vi "Func-엑셀 데이터를 그래프로 출력.vi"() -> ()   [LabVIEW 2015] (continued)
\t65\t69.654\n65\t65\t69.656\n65\t65\t69.657\n65\t65\t69.656\n65\t65\t69.656\n65\t65\t69.657\n65\t65\t69.658\n65\t65\t69.662\n65\t65\t69.662\n65\t65\t69.666\n65\t65\t69.667\n65\t65\t69.667\n65\t65\t69.668\n65\t65\t69.664\n65\t65\t69.666\n65\t65\t69.667\n65\t65\t69.671\n65\t65\t69.671\n65\t65\t69.671\n65\t65\t69.672\n65\t65\t69.675\n65\t65\t69.676\n65\t65\t69.675\n65\t65\t69.681\n65\t65\t69.685\n65\t65\t69.686\n65\t65\t69.688\n65\t65\t69.689\n65\t65\t69.69\n65\t65\t69.687\n65\t65\t69.687\n65\t65\t69.693\n65\t65\t69.694\n65\t65\t69.694\n65\t65\t69.696\n65\t65\t69.696\n65\t65\t69.699\n65\t65\t69.697\n65\t65\t69.696\n65\t65\t69.699\n65\t65\t69.695\n65\t65\t69.694\n65\t65\t69.693\n65\t65\t69.696\n65\t65\t69.698\n65\t65\t69.7\n65\t65\t69.707\n65\t65\t69.712\n65\t65\t69.717\n65\t65\t69.718\n65\t65\t69.72\n65\t65\t69.72\n65\t65\t69.719\n65\t65\t69.72\n65\t65\t69.721\n65\t65\t69.721\n65\t65\t69.722\n65\t65\t69.718\n65\t65\t69.721\n65\t65\t69.721\n65\t65\t69.719\n65\t65\t69.719\n65\t65\t69.718\n65\t65\t69.721\n65\t65\t69.725\n65\t65\t69.727\n65\t65\t69.73\n65\t65\t69.73\n65\t65\t69.73\n65\t65\t69.736\n65\t65\t69.736\n65\t65\t69.737\n65\t65\t69.739\n65\t65\t69.744\n65\t65\t69.746\n65\t65\t69.742\n65\t65\t69.743\n65\t65\t69.742\n65\t65\t69.746\n65\t65\t69.742\n65\t65\t69.746\n65\t65\t69.747\n65\t65\t69.751\n65\t65\t69.755\n65\t65\t69.755\n65\t65\t69.757\n65\t65\t69.761\n65\t65\t69.766\n65\t65\t69.764\n65\t65\t69.765\n65\t65\t69.763\n65\t65\t69.77\n65\t65\t69.771\n65\t65\t69.769\n65\t65\t69.773\n65\t65\t69.769\n65\t65\t69.771\n65\t65\t69.769\n65\t65\t69.766\n65\t65\t69.768\n65\t65\t69.768\n65\t65\t69.77\n65\t65\t69.772\n65\t65\t69.773\n65\t65\t69.773\n65\t65\t69.772\n65\t65\t69.773\n65\t65\t69.779\n65\t65\t69.78\n65\t65\t69.781\n65\t65\t69.786\n65\t65\t69.79\n65\t65\t69.793\n65\t65\t69.791\n65\t65\t69.789\n65\t65\t69.787\n65\t65\t69.788\n65\t65\t69.786\n65\t65\t69.784\n65\t65\t69.788\n65\t65\t69.79\n65\t65\t69.791\n65\t65\t69.79\n65\t65\t69.79\n65\t65\t69.792\n65\t65\t69.791\n65\t65\t69.789\n65\t65\t69.79\n65\t65\t69.795\n65\t65\t69.798\n65\t65\t69.8\n65\t65\t69.804\n65\t65\t69.806\n65\t65\t69.805\n65\t65\t69.803\n65\t65\t69.806\n65\t65\t69.806\n65\t65\t69.804\n65\t65\t69.808\n65\t65\t69.809\n65\t65\t69.81\n65\t65\t69.807\n65\t65\t69.809\n65\t65\t69.812\n65\t65\t69.811\n65\t65\t69.813\n65\t65\t69.816\n65\t65\t69.82\n65\t65\t69.821\n65\t65\t69.82\n65\t65\t69.823\n65\t65\t69.823\n65\t65\t69.826\n65\t65\t69.823\n65\t65\t69.824\n65\t65\t69.828\n65\t65\t69.832\n65\t65\t69.835\n65\t65\t69.833\n65\t65\t69.838\n65\t65\t69.838\n65\t65\t69.836\n65\t65\t69.833\n65\t65\t69.836\n65\t65\t69.836\n65\t65\t69.839\n65\t65\t69.843\n65\t65\t69.844\n65\t65\t69.85\n65\t65\t69.846\n65\t65\t69.847\n65\t65\t69.844\n65\t65\t69.845\n65\t65\t69.848\n65\t65\t69.844\n65\t65\t69.848\n65\t65\t69.852\n65\t65\t69.857\n65\t65\t69.855\n65\t65\t69.855\n65\t65\t69.86\n65\t65\t69.861\n65\t65\t69.857\n65\t65\t69.857\n65\t65\t69.859\n65\t65\t69.858\n65\t65\t69.856\n65\t65\t69.855\n65\t65\t69.856\n65\t65\t69.854\n65\t65\t69.854\n65\t65\t69.855\n65\t65\t69.858\n65\t65\t69.863\n65\t65\t69.868\n65\t65\t69.87\n65\t65\t69.873\n65\t65\t69.877\n65\t65\t69.875\n65\t65\t69.878\n65\t65\t69.879\n65\t65\t69.879\n65\t65\t69.877\n65\t65\t69.877\n65\t65\t69.877\n65\t65\t69.875\n65\t65\t69.874\n65\t65\t69.876\n65\t65\t69.877\n65\t65\t69.879\n65.083\t65.06\t70.457\n65.167\t65.12\t70.467\n65.25\t65.04\t70.467\n65.333\t64.94\t70.484\n65.417\t64.87\t70.475\n65.5\t64.77\t70.48\n65.583\t64.66\t70.477\n65.667\t64.54\t70.491\n65.75\t64.44\t70.489\n65.833\t64.34\t70.495\n65.917\t64.26\t70.497\n66\t64.18\t70.494\n66.083\t64.15\t70.494\n66.167\t64.12\t70.506\n66.25\t64.13\t70.493\n66.333\t64.15\t70.499\n66.417\t64.19\t70.495\n66.5\t64.25\t70.502\n66.583\t64.33\t70.495\n66.667\t64.42\t70.505\n66.75\t64.52\t70.501\n66.833\t64.63\t70.495\n66.917\t64.76\t70.491\n67\t64.89\t70.501\n67.083\t65.01\t70.506\n67.167\t65.14\t70.499\n67.25\t65.27\t70.494\n67.333\t65.4\t70.482\n67.417\t65.52\t70.498\n67.5\t65.64\t70.502\n67.583\t65.75\t70.504\n67.667\t65.85\t70.494\n67.75\t65.94\t70.503\n67.833\t66.03\t70.493\n67.917\t66.12\t70.498\n68\t66.21\t70.496\n68.083\t66.3\t70.507\n68.167\t66.38\t70.51\n68.25\t66.44\t70.51\n68.333\t66.52\t70.518\n68.417\t66.6\t70.514\n68.5\t66.67\t70.516\n68.583\t66.74\t70.525\n68.667\t66.81\t70.535\n68.75\t66.88\t70.533\n68.833\t66.95\t70.542\n68.917\t67.02\t70.544\n69\t67.1\t70.551\n69.083\t67.17\t70.559\n69.167\t67.24\t70.577\n69.25\t67.32\t70.583\n69.333\t67.4\t70.588\n69.417\t67.48\t70.612\n69.5\t67.56\t70.616\n69.583\t67.65\t70.624\n69.667\t67.73\t70.634\n69.75\t67.82\t70.644\n69.833\t67.9\t70.655\n69.917\t67.99\t70.665\n70\t68.07\t70.691\n70.083\t68.16\t70.706\n70.167\t68.25\t70.709\n70.25\t68.33\t70.732\n70.333\t68.41\t70.75\n70.417\t68.49\t70.766\n70.5\t68.57\t70.788\n70.583\t68.65\t70.798\n70.667\t68.72\t70.818\n70.75\t68.79\t70.832\n70.833\t68.87\t70.861\n70.917\t68.94\t70.886\n71\t69.01\t70.899\n71.083\t69.08\t70.924\n71.167\t69.15\t70.942\n71.25\t69.23\t70.965\n71.333\t69.31\t70.995\n71.417\t69.4\t71.013\n71.5\t69.47\t71.041\n71.583\t69.55\t71.06\n71.667\t69.63\t71.091\n71.75\t69.72\t71.109\n71.833\t69.79\t71.137\n71.917\t69.87\t71.155\n72\t69.96\t71.191\n72.083\t70.04\t71.219\n72.167\t70.12\t71.246\n72.25\t70.21\t71.273\n72.333\t70.28\t71.305\n72.417\t70.35\t71.341\n72.5\t70.43\t71.368\n72.583\t70.52\t71.398\n72.667\t70.6\t71.431\n72.75\t70.68\t71.465\n72.833\t70.75\t71.491\n72.917\t70.85\t71.529\n73\t70.95\t71.562\n73.083\t71.03\t71.589\n73.167\t71.1\t71.629\n73.25\t71.18\t71.661\n73.333\t71.26\t71.695\n73.417\t71.35\t71.732\n73.5\t71.44\t71.762\n73.583\t71.51\t71.796\n73.667\t71.6\t71.842\n73.75\t71.68\t71.891\n73.833\t71.77\t71.914\n73.917\t71.85\t71.955\n74\t71.95\t71.99\n74.083\t72.03\t72.033\n74.167\t72.12\t72.076\n74.25\t72.2\t72.118\n74.333\t72.28\t72.155\n74.417\t72.36\t72.19\n74.5\t72.45\t72.229\n74.583\t72.54\t72.275\n74.667\t72.62\t72.317\n74.75\t72.71\t72.354\n74.833\t72.79\t72.4\n74.917\t72.88\t72.451\n75\t72.97\t72.485\n75.083\t73.05\t72.525\n75.167\t73.14\t72.57\n75.25\t73.23\t72.625\n75.333\t73.32\t72.676\n75.417\t73.39\t72.714\n75.5\t73.48\t72.757\n75.583\t73.56\t72.803\n75.667\t73.64\t72.859\n75.75\t73.71\t72.902\n75.833\t73.8\t72.946\n75.917\t73.87\t72.994\n76\t73.95\t73.047\n76.083\t74.04\t73.093\n76.167\t74.12\t73.138\n76.25\t74.19\t73.19\n76.333\t74.29\t73.231\n76.417\t74.36\t73.286\n76.5\t74.43\t73.338\n76.583\t74.5\t73.391\n76.667\t74.58\t73.448\n76.75\t74.67\t73.487\n76.833\t74.73\t73.552\n76.917\t74.81\t73.599\n77\t74.89\t73.645\n77.083\t74.96\t73.697\n77.167\t75.03\t73.747\n77.25\t75.13\t73.803\n77.333\t75.22\t73.861\n77.417\t75.31\t73.913\n77.5\t75.39\t73.964\n77.583\t75.47\t74.02\n77.667\t75.56\t74.083\n77.75\t75.64\t74.129\n77.833\t75.75\t74.178\n77.917\t75.83\t74.235\n78\t75.92\t74.289\n78.083\t76.01\t74.354\n78.167\t76.09\t74.406\n78.25\t76.19\t74.462\n78.333\t76.27\t74.521\n78.417\t76.36\t74.575\n78.5\t76.44\t74.633\n78.583\t76.53\t74.685\n78.667\t76.61\t74.745\n78.75\t76.7\t74.807\n78.833\t76.78\t74.876\n78.917\t76.86\t74.925\n79\t76.93\t74.988\n79.083\t77.01\t75.031\n79.167\t77.1\t75.092\n79.25\t77.17\t75.159\n79.333\t77.25\t75.212\n79.417\t77.32\t75.278\n79.5\t77.38\t75.335\n79.583\t77.46\t75.405\n79.667\t77.55\t75.454\n79.75\t77.63\t75.521\n79.833\t77.7\t75.579\n79.917\t77.78\t75.64\n80\t77.87\t75.699\n80.083\t77.95\t75.763\n80.167\t78.04\t75.835\n80.25\t78.13\t75.897\n80.333\t78.21\t75.958\n80.417\t78.28\t76.013\n80.5\t78.35\t76.079\n80.583\t78.42\t76.156\n80.667\t78.51\t76.198\n80.75\t78.59\t76.271\n80.833\t78.66\t76.334\n80.917\t78.74\t76.404\n81\t78.82\t76.461\n81.083\t78.9\t76.53\n81.167\t78.99\t76.588\n81.25\t79.08\t76.653\n81.333\t79.16\t76.718\n81.417\t79.23\t76.778\n81.5\t79.32\t76.851\n81.583\t79.4\t76.918\n81.667\t79.49\t76.985\n81.75\t79.57\t77.039\n81.833\t79.65\t77.109\n81.917\t79.74\t77.178\n82\t79.81\t77.242\n82.083\t79.91\t77.295\n82.167\t79.99\t77.368\n82.25\t80.08\t77.443\n82.333\t80.15\t77.496\n82.417\t80.24\t77.565\n82.5\t80.33\t77.635\n82.583\t80.41\t77.704\n82.667\t80.48\t77.763\n82.75\t80.56\t77.827\n82.833\t80.66\t77.901\n82.917\t80.74\t77.966\n83\t80.81\t78.036\n83.083\t80.9\t78.098\n83.167\t80.99\t78.164\n83.25\t81.06\t78.234\n83.333\t81.14\t78.297\n83.417\t81.22\t78.361\n83.5\t81.31\t78.441\n83.583\t81.4\t78.506\n83.667\t81.49\t78.576\n83.75\t81.57\t78.64\n83.833\t81.66\t78.698\n83.917\t81.73\t78.78\n84\t81.81\t78.841\n84.083\t81.89\t78.913\n84.167\t81.96\t78.985\n84.25\t82.04\t79.053\n84.333\t82.11\t79.114\n84.417\t82.17\t79.187\n84.5\t82.26\t79.259\n84.583\t82.35\t79.32\n84.667\t82.43\t79.391\n84.75\t82.51\t79.466\n84.833\t82.6\t79.528\n84.917\t82.69\t79.601\n85\t82.76\t79.662\n85\t82.77\t79.665\n85\t82.78\t79.667\n85\t82.79\t79.671\n85\t82.8\t79.673\n85\t82.81\t79.68\n85\t82.82\t79.688\n85\t82.82\t79.696\n85\t82.82\t79.709\n85\t82.83\t79.716\n85\t82.84\t79.724\n85\t82.85\t79.737\n85\t82.86\t79.741\n85\t82.86\t79.747\n85\t82.87\t79.755\n85\t82.88\t79.764\n85\t82.89\t79.775\n85\t82.9\t79.783\n85\t82.91\t79.791\n85\t82.91\t79.801\n85\t82.92\t79.808\n85\t82.93\t79.813\n85\t82.93\t79.818\n85\t82.94\t79.826\n85\t82.95\t79.831\n85\t82.96\t79.835\n85\t82.97\t79.84\n85\t82.97\t79.845\n85\t82.98\t79.854\n85\t82.99\t79.855\n85\t83\t79.863\n85\t83.01\t79.874\n85\t83.02\t79.879\n85\t83.03\t79.883\n85\t83.03\t79.896\n85\t83.04\t79.91\n85\t83.04\t79.913\n85\t83.05\t79.921\n85\t83.06\t79.928\n85\t83.07\t79.933\n85\t83.07\t79.941\n85\t83.08\t79.945\n85\t83.09\t79.954\n85\t83.1\t79.961\n85\t83.11\t79.967\n85\t83.12\t79.974\n85\t83.13\t79.975\n85\t83.14\t79.981\n85\t83.14\t79.99\n85\t83.15\t79.994\n85\t83.15\t80.003\n85\t83.15\t80.014\n85\t83.15\t80.022\n85\t83.16\t80.028\n85\t83.17\t80.038\n85\t83.18\t80.048\n85\t83.19\t80.052\n85\t83.2\t80.064\n85\t83.2\t80.071\n85\t83.21\t80.078\n85\t83.21\t80.082\n85\t83.22\t80.085\n85\t83.22\t80.096\n85\t83.23\t80.098\n85\t83.23\t80.104\n85\t83.24\t80.113\n85\t83.24\t80.118\n85\t83.25\t80.125\n85\t83.25\t80.132\n85\t83.25\t80.139\n85\t83.25\t80.146\n85\t83.26\t80.159\n85\t83.27\t80.165\n85\t83.27\t80.17\n85\t83.28\t80.183\n85\t83.29\t80.189\n85\t83.29\t80.196\n85\t83.3\t80.199\n85\t83.3\t80.208\n85\t83.31\t80.214\n85\t83.31\t80.217\n85\t83.32\t80.221\n85\t83.33\t80.229\n85\t83.33\t80.234\n85\t83.34\t80.242\n85\t83.35\t80.252\n85\t83.36\t80.259\n85\t83.36\t80.268\n85\t83.36\t80.274\n85\t83.36\t80.281\n85\t83.36\t80.286\n85\t83.37\t80.291\n85\t83.38\t80.298\n85\t83.39\t80.304\n85\t83.39\t80.315\n85\t83.4\t80.319\n85\t83.41\t80.331\n85\t83.41\t80.337\n85\t83.41\t80.343\n85\t83.42\t80.35\n85\t83.42\t80.355\n85\t83.43\t80.365\n85\t83.44\t80.371\n85\t83.45\t80.377\n85\t83.45\t80.386\n85\t83.46\t80.395\n85\t83.46\t80.401\n85\t83.47\t80.405\n85\t83.47\t80.416\n85\t83.47\t80.427\n85\t83.47\t80.429\n85\t83.47\t80.434\n85\t83.47\t80.442\n85\t83.48\t80.455\n85\t83.48\t80.456\n85\t83.49\t80.459\n85\t83.5\t80.473\n85\t83.5\t80.481\n85\t83.5\t80.488\n85\t83.51\t80.494\n85\t83.52\t80.502\n85\t83.52\t80.509\n85\t83.53\t80.516\n85\t83.54\t80.518\n85\t83.54\t80.522\n85\t83.55\t80.527\n85\t83.55\t80.536\n85\t83.56\t80.54\n85\t83.57\t80.548\n85\t83.58\t80.56\n85\t83.58\t80.568\n85\t83.58\t80.575\n85\t83.58\t80.58\n85\t83.59\t80.591\n85\t83.59\t80.594\n85\t83.6\t80.599\n85\t83.61\t80.607\n85\t83.61\t80.619\n85\t83.62\t80.624\n85\t83.63\t80.63\n85\t83.64\t80.636\n85\t83.65\t80.639\n85\t83.65\t80.646\n85\t83.66\t80.649\n85\t83.67\t80.655\n85\t83.68\t80.667\n85\t83.68\t80.676\n85\t83.69\t80.684\n85\t83.69\t80.694\n85\t83.69\t80.702\n85\t83.69\t80.712\n85\t83.69\t80.716\n85\t83.7\t80.72\n85\t83.71\t80.729\n85\t83.71\t80.735\n85\t83.72\t80.736\n85\t83.73\t80.741\n85\t83.73\t80.748\n85\t83.74\t80.754\n85\t83.75\t80.764\n85\t83.75\t80.771\n85\t83.76\t80.782\n85\t83.77\t80.793\n85\t83.77\t80.801\n85\t83.78\t80.811\n85\t83.79\t80.815\n85\t83.8\t80.82\n85\t83.8\t80.826\n85\t83.8\t80.834\n85\t83.81\t80.84\n85\t83.82\t80.845\n85\t83.82\t80.852\n85\t83.83\t80.859\n85\t83.84\t80.864\n85\t83.84\t80.871\n85\t83.85\t80.879\n85\t83.86\t80.888\n85\t83.87\t80.895\n85\t83.88\t80.9\n85\t83.89\t80.91\n85\t83.89\t80.919\n85\t83.9\t80.921\n85\t83.91\t80.93\n85\t83.91\t80.936\n85\t83.91\t80.944\n85\t83.92\t80.953\n85\t83.93\t80.958\n85\t83.94\t80.967\n85\t83.95\t80.974\n85\t83.95\t80.982\n85\t83.96\t80.987\n85\t83.97\t80.993\n85\t83.98\t80.996\n85\t83.99\t81.004\n85\t84\t81.007\n85\t84\t81.013\n85\t84.01\t81.023\n85\t84.01\t81.032\n85\t84.02\t81.038\n85\t84.02\t81.054\n85\t84.03\t81.064\n85\t84.03\t81.071\n85\t84.04\t81.076\n85\t84.04\t81.083\n85\t84.05\t81.095\n85\t84.06\t81.097\n85\t84.06\t81.105\n85\t84.07\t81.111\n85\t84.08\t81.121\n85\t84.09\t81.126\n85\t84.09\t81.129\n85\t84.1\t81.133\n85\t84.11\t81.136\n85\t84.11\t81.146\n85\t84.12\t81.154\n85\t84.12\t81.157\n85\t84.12\t81.168\n85\t84.13\t81.177\n85\t84.14\t81.186\n85\t84.14\t81.193\n85\t84.15\t81.201\n85\t84.15\t81.213\n85\t84.16\t81.218\n85\t84.16\t81.226\n85\t84.17\t81.227\n85\t84.17\t81.232\n85\t84.18\t81.238\n85\t84.18\t81.246\n85\t84.19\t81.254\n85\t84.2\t81.261\n85\t84.2\t81.273\n85\t84.21\t81.282\n85\t84.22\t81.286\n85\t84.22\t81.292\n85\t84.23\t81.3\n85\t84.23\t81.303\n85\t84.23\t81.314\n85\t84.24\t81.319\n85\t84.24\t81.325\n85\t84.25\t81.336\n85\t84.25\t81.345\n85\t84.26\t81.35\n85\t84.26\t81.358\n85\t84.27\t81.364\n85\t84.28\t81.37\n85\t84.28\t81.378\n85\t84.29\t81.384\n85\t84.3\t81.398\n85\t84.3\t81.405\n85\t84.3\t81.416\n85\t84.31\t81.422\n85\t84.32\t81.427\n85\t84.32\t81.431\n85\t84.33\t81.436\n85\t84.34\t81.443\n85\t84.34\t81.442\n85\t84.34\t81.453\n85\t84.35\t81.457\n85\t84.36\t81.461\n85\t84.36\t81.466\n85\t84.37\t81.47\n85\t84.38\t81.479\n85\t84.38\t81.486\n85\t84.39\t81.491\n85\t84.39\t81.502\n85\t84.4\t81.509\n85\t84.41\t81.516\n85\t84.42\t81.523\n85\t84.43\t81.53\n85\t84.43\t81.539\n85\t84.44\t81.549\n85\t84.44\t81.555\n85\t84.45\t81.56\n85\t84.45\t81.566\n85\t84.45\t81.572\n85\t84.46\t81.579\n85\t84.46\t81.589\n85\t84.47\t81.6\n85\t84.47\t81.61\n85\t84.47\t81.617\n85\t84.48\t81.628\n85\t84.48\t81.629\n85\t84.49\t81.635\n85\t84.49\t81.638\n85\t84.5\t81.648\n85\t84.5\t81.657\n85\t84.51\t81.662\n85\t84.51\t81.676\n85\t84.51\t81.68\n85\t84.52\t81.687\n85\t84.52\t81.695\n85\t84.53\t81.7\n85\t84.53\t81.7\n85\t84.54\t81.705\n85\t84.55\t81.714\n85\t84.55\t81.722\n85\t84.55\t81.724\n85\t84.55\t81.729\n85\t84.56\t81.742\n85\t84.56\t81.748\n85\t84.56\t81.755\n85\t84.56\t81.764\n85\t84.57\t81.773\n85\t84.57\t81.776\n85\t84.57\t81.786\n85\t84.58\t81.789\n85\t84.58\t81.793\n85\t84.59\t81.8\n85\t84.59\t81.804\n85\t84.59\t81.81\n85\t84.59\t81.816\n85\t84.6\t81.829\n85\t84.6\t81.839\n85\t84.61\t81.849\n85\t84.61\t81.857\n85\t84.61\t81.871\n85\t84.61\t81.877\n85\t84.61\t81.881\n85\t84.61\t81.89\n85\t84.61\t81.893\n85\t84.62\t81.899\n85\t84.62\t81.909\n85\t84.62\t81.916\n85\t84.62\t81.92\n85\t84.63\t81.931\n85\t84.63\t81.934\n85\t84.63\t81.941\n85\t84.63\t81.948\n85\t84.64\t81.953\n85\t84.64\t81.962\n85\t84.64\t81.968\n85\t84.64\t81.978\n85\t84.64\t81.986\n85\t84.64\t81.993\n85\t84.65\t81.999\n85\t84.65\t82.005\n85\t84.65\t82.016\n85\t84.65\t82.018\n85\t84.65\t82.023\n85\t84.66\t82.03\n85\t84.66\t82.037\n85\t84.66\t82.043\n85\t84.66\t82.047\n85\t84.67\t82.058\n85\t84.67\t82.068\n85\t84.67\t82.075\n85\t84.67\t82.08\n85\t84.67\t82.089\n85\t84.67\t82.093\n85\t84.67\t82.098\n85\t84.67\t82.109\n85\t84.68\t82.114\n85\t84.68\t82.123\n85\t84.68\t82.13\n85\t84.69\t82.138\n85\t84.69\t82.144\n85\t84.69\t82.148\n85\t84.7\t82.153\n85\t84.7\t82.167\n85\t84.7\t82.173\n85\t84.7\t82.18\n85\t84.71\t82.191\n85\t84.71\t82.196\n85\t84.71\t82.203\n85\t84.71\t82.207\n85\t84.71\t82.213\n85\t84.72\t82.218\n85\t84.72\t82.226\n85\t84.72\t82.232\n85\t84.73\t82.238\n85\t84.73\t82.247\n85\t84.73\t82.253\n85\t84.74\t82.261\n85\t84.74\t82.266\n85\t84.74\t82.274\n85\t84.75\t82.285\n85\t84.75\t82.288\n85\t84.76\t82.291\n85\t84.76\t82.302\n85\t84.77\t82.307\n85\t84.77\t82.313\n85\t84.77\t82.314\n85\t84.77\t82.318\n85\t84.78\t82.326\n85\t84.78\t82.335\n85\t84.78\t82.343\n85\t84.78\t82.35\n85\t84.78\t82.363\n85\t84.78\t82.37\n85\t84.79\t82.379\n85\t84.8\t82.384\n85\t84.8\t82.39\n85\t84.8\t82.396\n85\t84.81\t82.405\n85\t84.81\t82.413\n85\t84.81\t82.422\n85\t84.81\t82.429\n85\t84.81\t82.435\n85\t84.82\t82.439\n85\t84.82\t82.449\n85\t84.82\t82.456\n85\t84.83\t82.458\n85\t84.83\t82.463\n85\t84.82\t82.467\n85\t84.83\t82.477\n85\t84.83\t82.484\n85\t84.83\t82.489\n85\t84.83\t82.501\n85\t84.84\t82.511\n85\t84.84\t82.519\n85\t84.84\t82.531\n85\t84.85\t82.533\n85\t84.85\t82.545\n85\t84.85\t82.552\n85\t84.85\t82.555\n85\t84.85\t82.567\n85\t84.86\t82.57\n85\t84.86\t82.577\n85\t84.86\t82.58\n85\t84.87\t82.581\n85\t84.87\t82.591\n85\t84.87\t82.594\n85\t84.88\t82.601\n85\t84.88\t82.604\n85\t84.88\t82.618\n85\t84.88\t82.628\n85\t84.88\t82.629\n85\t84.88\t82.638\n85\t84.88\t82.648\n85\t84.88\t82.658\n85\t84.88\t82.658\n85\t84.88\t82.666\n85\t84.88\t82.675\n85\t84.89\t82.682\n85\t84.9\t82.686\n85\t84.91\t82.688\n85\t84.92\t82.696\n85\t84.93\t82.701\n85\t84.94\t82.707\n85\t84.95\t82.713\n85\t84.96\t82.716\n85\t84.97\t82.729\n85\t84.98\t82.736\n85\t85\t82.744\n85\t84.97\t82.751\n85\t84.97\t82.756\n85\t84.97\t82.766\n85\t84.97\t82.773\n85\t84.97\t82.781\n85\t84.97\t82.789\n85\t84.97\t82.795\n85\t84.97\t82.805\n85\t84.97\t82.811\n85\t84.97\t82.816\n85\t84.97\t82.819\n85\t84.97\t82.832\n85\t84.97\t82.836\n85\t84.97\t82.839\n85\t84.97\t82.846\n85\t84.97\t82.851\n85\t84.97\t82.857\n85\t84.97\t82.86\n85\t84.97\t82.871\n85\t84.97\t82.883\n85\t84.97\t82.89\n85\t84.97\t82.895\n85\t84.97\t82.904\n85\t84.97\t82.905\n85\t84.97\t82.911\n85\t84.97\t82.917\n85\t84.97\t82.923\n85\t84.97\t82.934\n85\t84.97\t82.942\n85\t84.97\t82.948\n85\t84.97\t82.95\n85\t84.97\t82.961\n85\t84.97\t82.966\n85\t84.97\t82.971\n85\t84.97\t82.978\n85\t84.98\t82.986\n85\t84.98\t82.999\n85\t84.98\t83.003\n85\t84.98\t83.009\n85\t84.98\t83.016\n85\t84.98\t83.021\n85\t84.98\t83.029\n85\t84.98\t83.032\n85\t84.98\t83.034\n85\t84.98\t83.042\n85\t84.98\t83.053\n85\t84.98\t83.057\n85\t84.98\t83.062\n85\t84.98\t83.07\n85\t84.98\t83.079\n85\t84.98\t83.085\n85\t84.98\t83.094\n85\t84.98\t83.105\n85\t84.98\t83.108\n85\t84.98\t83.117\n85\t84.98\t83.124\n85\t84.98\t83.129\n85\t84.98\t83.131\n85\t84.98\t83.135\n85\t84.98\t83.145\n85\t84.98\t83.151\n85\t84.98\t83.156\n85\t84.98\t83.168\n85\t84.98\t83.174\n85\t84.98\t83.182\n85\t84.98\t83.188\n85\t84.98\t83.193\n85\t84.98\t83.204\n85\t84.98\t83.213\n85\t84.98\t83.222\n85\t84.98\t83.222\n85\t84.98\t83.23\n85\t84.98\t83.236\n85\t84.98\t83.238\n85\t84.98\t83.239\n85\t84.98\t83.243\n85\t84.98\t83.257\n85\t84.98\t83.265\n85\t84.98\t83.274\n85\t84.98\t83.282\n85\t85\t83.291\n85\t85\t83.293\n85\t85\t83.298\n85\t85\t83.304\n85\t85\t83.311\n85\t85\t83.321\n85\t85\t83.326\n85\t85\t83.336\n85\t85\t83.345\n85\t85\t83.348\n85\t85\t83.352\n85\t85\t83.357\n85\t85\t83.361\n85\t85\t83.369\n85\t85\t83.372\n85\t85\t83.379\n85\t85\t83.387\n85\t85\t83.389\n85\t85\t83.394\n85\t85\t83.4\n85\t85\t83.408\n85\t85\t83.416\n85\t85\t83.421\n85\t85\t83.43\n85\t85\t83.44\n85\t85\t83.441\n85\t85\t83.444\n85\t85\t83.452\n85\t85\t83.46\n85\t85\t83.467\n85\t85\t83.477\n85\t85\t83.485\n85\t85\t83.491\n85\t85\t83.496\n85\t85\t83.502\n85\t85\t83.509\n85\t85\t83.518\n85\t85\t83.524\n85\t85\t83.53\n85\t85\t83.539\n85\t85\t83.543\n85\t85\t83.547\n85\t85\t83.552\n85\t85\t83.558\n85\t85\t83.566\n85\t85\t83.575\n85\t85\t83.586\n85\t85\t83.594\n85\t85\t83.597\n85\t85\t83.605\n85\t85\t83.61\n85\t85\t83.613\n85\t85\t83.615\n85\t85\t83.626\n85\t85\t83.631\n85\t85\t83.634\n85\t85\t83.641\n85\t85\t83.645\n85\t85\t83.648\n85\t85\t83.655\n85\t85\t83.661\n85\t85\t83.668\n85\t85\t83.677\n85\t85\t83.682\n85\t85\t83.696\n85\t85\t83.702\n85\t85\t83.706\n85\t85\t83.711\n85\t85\t83.718\n85\t85\t83.729\n85\t85\t83.739\n85\t85\t83.74\n85\t85\t83.751\n85\t85\t83.76\n85\t85\t83.763\n85\t85\t83.767\n85\t85\t83.77\n85\t85\t83.779\n85\t85\t83.785\n85\t85\t83.791\n85\t85\t83.793\n85\t85\t83.798\n85\t85\t83.804\n85\t85\t83.809\n85\t85\t83.814\n85\t85\t83.822\n85\t85\t83.831\n85\t85\t83.843\n85\t85\t83.85\n85\t85\t83.851\n85\t85\t83.862\n85\t85\t83.867\n85\t85\t83.871\n85\t85\t83.873\n85\t85\t83.877
